vi "FC2.vi"() -> ()   [LabVIEW 2017]
uses:
  BERTTA.dll
panel:
  out "element 2":i32
  out "element":i32
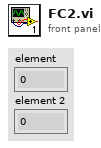
[diagram p1: front panel]
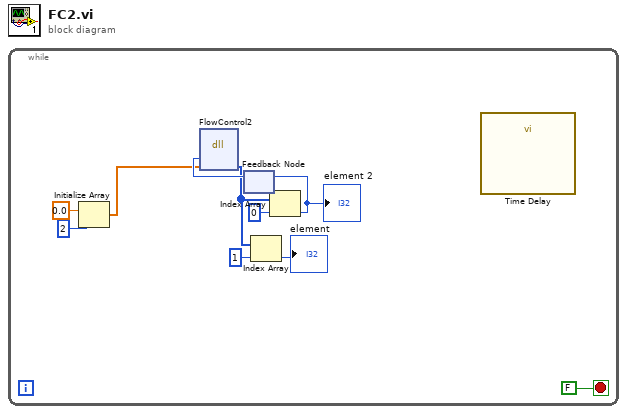
[diagram p0: block diagram]
diagram:
  n1 = while {
    stop <- FALSE stop-if-true
    n2 = Initialize Array(0.0 ("element"), 2 ("dimension size")) -> (w6:dbl[])
    n3 = feedback #1() -> (w7:i32)  [unwired: 1 in]
    n4 = dll-call lib="C:/Users/p3cn/OneDrive - Kemira Oyj/Documents/GitHub/Bertta/BERTTA/x64/Release/BERTTA.dll" fn="FlowControl2"("lastTime"=w7, "params"=w6) -> ("params"=w3:i32[])  [unwired: 5 in, 2 out]
    n5 = Index Array(array=w3, index=1) -> (element=→"element":i32)
    n6 = Index Array(array=w3, index=0) -> (element=w8:i32)
    "element 2" <- w8
    n7 = feedback-in #1(w8) -> ()
    n8 = call "Time Delay"() -> ()  [unwired: 11 in, 1 out]
  }
